vi "复件 SIMCOMCommunicationTool.vi"(6 "Debug":bool=TRUE, 7 "MEID":string, 8 "error in":errorcluster, 9 "DelayTime":u32=100, 10 "通信协议名称":string, 11 "VISA资源名称":refnum<visa-resource-name>="COM26") -> (0 "error out":errorcluster, 1 "CMD":string="发送 重启:AT+CRESET\r反馈:\r\nOK\r\n\r\n", 2 "反馈结果":bool=TRUE, 3 "响应":string="\r\nOK\r\n", 4 "ReturnData":string)   [LabVIEW 2013]
doc: "本范例根据用户指示，对串口执行读写操作。范例运行时可按下“写入”或“读取”按钮，以及修改“读数”。\n\n设置的串口参数必须匹配连接仪器或设备的参数。本范例中，“读数”参数可指定串口读取的字节数。如端口字节超过指定的字节数，超出部分将不会被读取。如端口字节数少于指定的字节数，将返回超时错误。\n\n本范例可扩展流控制选项以包括XON和XOFF，从而允许用户选择控制字符。同时，用户可启用或禁用中止符。部分设备需要通过终止符确定命令字符串的结束位置。部分设备将发送终止符以说明待读取数据的末端。本范例演示了缓冲区中检测到终止符时，结束“读取”操作或添加终止符至“写入”数据末端的方法。"
uses:
  <vilib>/Utility/NIReport.llb/NI_report.lvclass
  C:/Program Files/National Instruments/LabVIEW 2013/examples/Instrument IO/Serial/support/Serial - Settings.ctl
  SourceCode/GlobalValue.vi
  <vilib>/Utility/error.llb/Error Cluster From Error Code.vi
  <vilib>/addons/_office/excel.llb/Excel Get Data ([str]).vi
  <vilib>/Instr/_visa.llb/VISA Configure Serial Port (Instr).vi
  <vilib>/ErrorRing/Error Ring.xnode
  <vilib>/addons/_office/NI_ReportGenerationToolkit.lvlib
  <vilib>/Utility/NIReport.llb/Excel/NI_Excel.lvclass
panel:
  out "Data":string[][](array[string])=[["8986031490021881534", "460036161669975", "2A645416CB435F94", "8006A127", "460036161669975@mycdma.cn", "DB60264368A1D188", "18101891253", "A1000021A59070"], ["8986031490021881535", "460036161669976", "32FA5764D69C76BE", "80FAE4E6", "460036161669976@mycdma.cn", "B3AA1B3D2F0D5593", "18964872399", "A1000021A58D61"], ["", "", "", "", "", "", "", ""], ["", "", "", "", "", "", "", ""], ["", "", "", "", "", "", "", ""], ["", "", "", "", "", "", "", ""], ["", "", "", "", "", "", "", ""], ["", "", "", "", "", "", "", ""], ["", "", "", "", "", "", "", ""], ["", "", "", "", "", "", "", ""], ["", "各位，模块烧号主要是写五码，包括IMSI、AKEY、MEID（ESN）、AN(EVDO USER)、AAA(EVDO PWD)。", "", "", "", "", "", ""], ["", "其中ESN和MEID在模块出厂时已经写入，两者均可通过AT指令读取，但ESN不可更改。", "", "", "", "", "", ""], ["", "经询问及实际测试，上海电信绑定ESN号而广东电信未绑定，意味着上海电信五码烧录到其它模块是不可用的，但广东电信则无此限制。", "", "", "", "", "", ""], ["", "", "", "", "", "", "", ""], ["", "", "", "", "", "", "", ""], ["", "目前已确定跟上海电信合作，后续模块及卡号使用过程中，如遇到模块损坏，则意味着该卡必须销号（除非向电信申请绑定新的ESN），否则烧录到其它模块中是没用的。", "", "", "", "", "", ""]]
  in  "命令列表":u16(ring)=18 items=["查询RTRECF", "设置RTRECF", "查询MEID", "设置MEID", "查询ESN", "设置ESN", "查询AKEY", "设置AKEY", "查询IMSI1", "设置IMSI1", "查询IMSI2", "设置IMSI2", "查询IMSI3", "设置IMSI3", "设置EVDO账号", "设置EVDO密码", "打开音频LOOPBACK", "关闭音频LOOPBACK", "重启"]
  out "ConfigPath":string="D:\\导航\\T-BOX\\新建文件夹\\config\\通信协议.xls"
  out "DataType":string="AT+CRESET"
  out "命令":string="AT+CRESET\r"
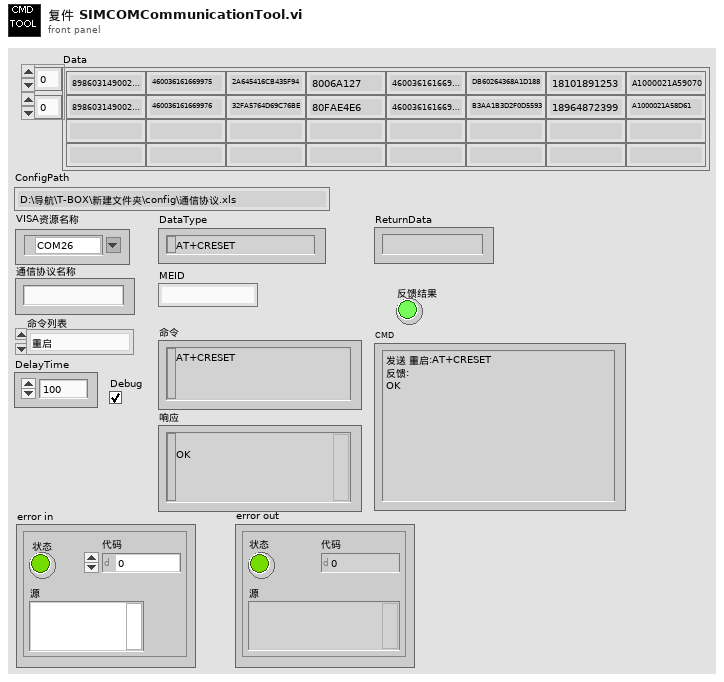
[diagram p1: front panel]
types:
  T1 = enum32{"invalid app kind", "Development System", "Run Time System", "Student Edition", "Embedded LabVIEW", "Evaluation", "Custom"}
  T2 = enum16{"maximized", "minimized", "normal", "no change"}
  T3 = enum16{"Standard Report", "HTML", "Word", "Excel"}
  T4 = typedef "Serial - Settings.ctl" = cluster{"波特率":u32, "数据比特":u16, "奇偶":enum16{"None", "Odd", "Even", "Mark", "Space"}, "停止位":u16, "流控制":u16}
  T5 = cluster{"IMSI":string, "AKEY":string, "ESN":string, "EVDO账号":string, "EVDO密码":string}
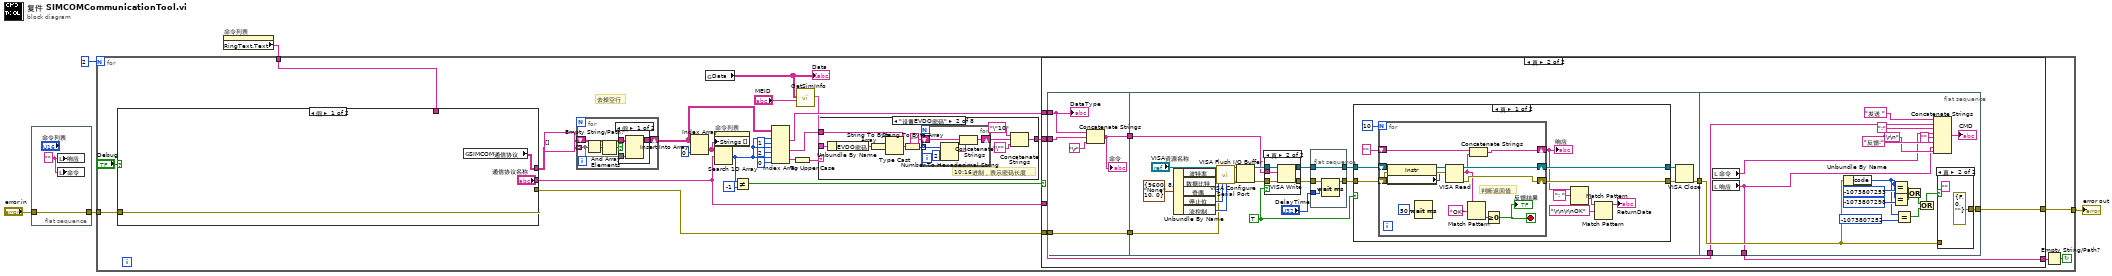
[diagram p0: block diagram]
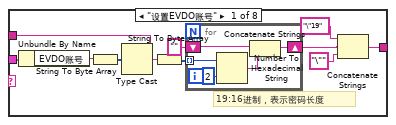
[diagram p3: hidden frame]
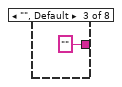
[diagram p4: hidden frame]
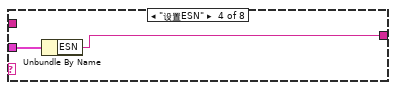
[diagram p5: hidden frame]
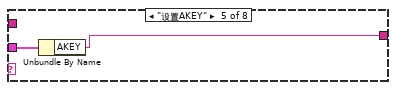
[diagram p6: hidden frame]
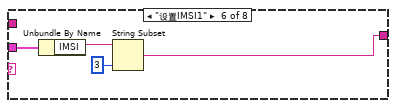
[diagram p7: hidden frame]
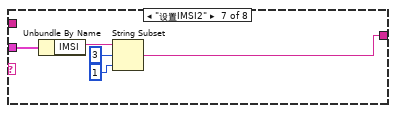
[diagram p8: hidden frame]
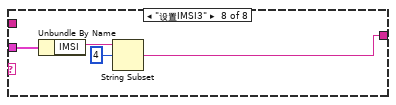
[diagram p9: hidden frame]
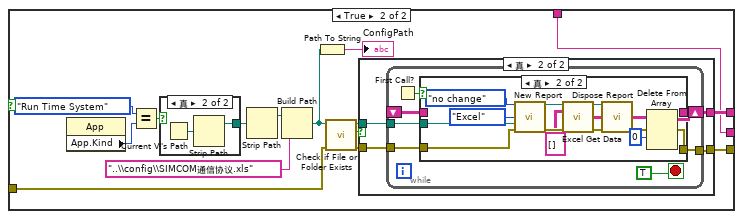
[diagram p10: hidden frame]
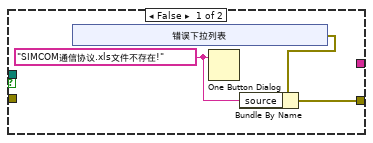
[diagram p11: hidden frame]
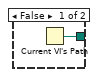
[diagram p13: hidden frame]
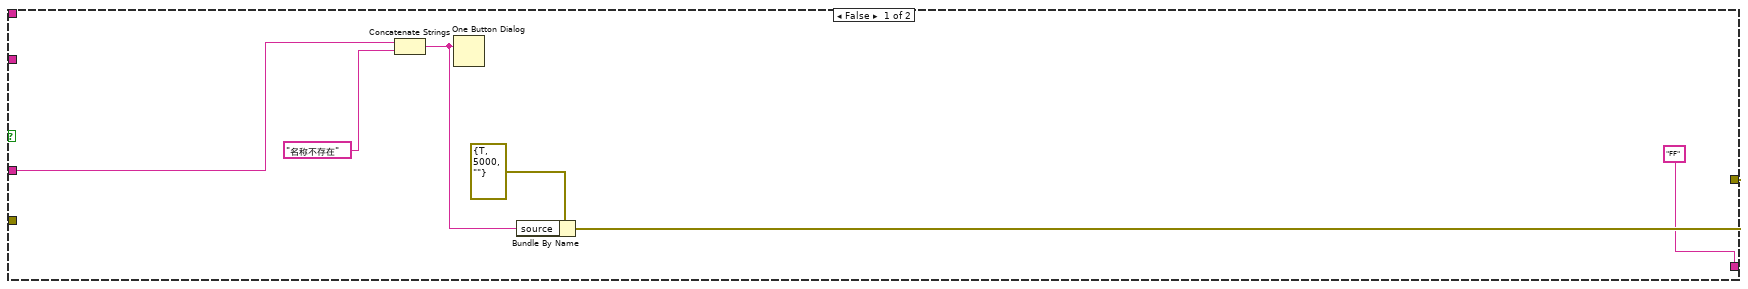
[diagram p14: hidden frame]
diagram:
  n1 = flat-sequence {
    tunnel: "error in" -> [w6]
    tunnel: [w6] -> w2
    frame #0 {
      w7 = "" ("响应")
      n2 = local write "响应"(w7) -> ()
      n3 = local write "命令"(w7) -> ()
    }
  }
  n4 = property on="命令列表" class="Ring (严格)"() -> ("RingText.Text"=w1:string)  [unwired: 2 in, 2 out]
  n5 = for {
    N: 2 -> [_]
    tunnel: w2 -> [w22]
    tunnel: [w34] -> w5
    tunnel: w1 -> [w14]
    stop <- w20 continue-if-true
    # "去掉空行"
    n6 = case shown="假" "Debug" {
      tunnel: [w93 w98] -> w33
      tunnel: w22 -> [w93 w97]
      tunnel: ["通信协议名称" w95] -> w26
      tunnel: [w92 w96] -> w16
      tunnel: w14 -> [_ w95]
      frame False {
        n7 = global read "GlobalValue.vi" "SIMCOM通信协议"() -> (w92:string[][])
      }
      frame True {
        n8 = property class="App"() -> ("App.Kind"=w107:T1)  [unwired: 2 in, 2 out]
        n9 = Equal?(x=T1."Run Time System" ("y"), y=w107) -> (x = y?=w109:bool)
        n10 = case shown="真" w109 {
          tunnel: [w143 w145] -> w108
          frame False {
            n11 = Current VI's Path() -> (path=w143:path)
          }
          frame True {
            n12 = Current VI's Path() -> (path=w144:path)
            n13 = Strip Path(path=w144) -> (stripped path=w145:path)  [unwired: 1 out]
          }
        }
        n14 = Strip Path(path=w108) -> (stripped path=w102:path)  [unwired: 1 out]
        n15 = Build Path(base path=w102, name or relative path="..\\config\\SIMCOM通信协议.xls" ("连接的字符串")) -> (appended path=w104:path)
        n16 = Path To String(path=w104) -> (string=→"ConfigPath":string)
        n17 = call <vilib>:"Check if File or Folder Exists.vi"("error in (no error)"=w97, "path"=w104) -> ("error out"=w99:errorcluster, "file or folder exists?"=w101:bool, "dup path"=w100:path)  [unwired: 7 out]
        n18 = case shown="真" w101 {
          tunnel: w100 -> [_ w120]
          tunnel: w99 -> [_ w119]
          tunnel: [w111 w118] -> w98
          tunnel: [_ w117] -> w96
          frame False {
            w112 = "SIMCOM通信协议.xls文件不存在!" ("消息")
            n19 = xnode "错误下拉列表"() -> ("错误输出"=w110:errorcluster)
            n20 = One Button Dialog(message=w112) -> ()  [unwired: 1 in, 1 out]
            n21 = Bundle By Name(cluster=w110, "source"=w112) -> (w111:errorcluster)
          }
          frame True {
            n22 = while {
              tunnel: w120 -> [w126]
              tunnel: [w125] -> w118
              tunnel: w119 -> [w124]
              shift-right: [w127] -> w117
              shift-left: _ -> [w122]
              stop <- TRUE stop-if-true
              n23 = First Call?() -> (First Call?: T/F=w121:bool)
              n24 = case shown="真" w121 {
                tunnel: [w129 w133] -> w127
                tunnel: w126 -> [_ w132]
                tunnel: [w128 w131] -> w125
                tunnel: w124 -> [w128 w130]
                tunnel: w122 -> [w129 _]
                frame False {
                }
                frame True {
                  n25 = call <vilib>:"New Report.vi"("window state (normal)"=T2."no change", "report type"=T3."Excel", "template (empty)"=w132, "error in (no error)"=w130) -> ("report out"=w138:refnum<class "NI_report.lvclass">, "error out"=w139:errorcluster)  [unwired: 2 in, 8 out]
                  n26 = call-poly <vilib>:"Excel Get Data.vi"("report in"=w138, "data type"=string[][] [], "error in (no error)"=w139) -> ("report out"=w135:refnum<class "NI_report.lvclass">, "data"=w140:string[][], "error out"=w134:errorcluster)  [unwired: 10 in]
                  n27 = call-dynamic "Dispose Report.vi"("report in"=w135, "error in (no error)"=w134) -> ("error out"=w131:errorcluster)  [unwired: 3 in, 10 out]
                  n28 = Delete From Array(array=w140, index (row)=0 ("索引 (行)")) -> (array with subset deleted=w133:string[][])  [unwired: 2 in, 1 out]
                }
              }
            }
          }
        }
      }
    }
    n29 = for {
      tunnel: w16 -> [w35] mode=indexing
      shift-right: [w38] -> w15
      shift-left: string[][] [] -> [w39]
      n30 = Empty String/Path?(string/path=w35) -> (empty?=w37:bool[])
      n31 = And Array Elements(Boolean array=w37) -> (logical AND=w36:bool)
      n32 = case shown="假" w36 {
        tunnel: w39 -> [w42 w43]
        tunnel: [w41 w43] -> w38
        tunnel: w35 -> [w40 _]
        frame False {
          n33 = Insert Into Array(array=w42, new element=w40) -> (w41:string[][])  [unwired: 2 in]
        }
        frame True {
        }
      }
    }
    n34 = Index Array(array=w15, index (col)=0 ("禁用的索引 (列)")) -> (element=w24:string[])  [unwired: 1 in]
    n35 = global read "GlobalValue.vi" "Data"() -> (w9:string[][])
    "Data" <- w9
    n36 = property on="命令列表" class="Ring (严格)"("Strings []"=w24) -> ()  [unwired: 2 in, 2 out]
    n37 = Search 1D Array(1D array=w24, element=w26) -> (index of element=w19:i32)  [unwired: 1 in]
    n38 = Not Equal?(x=w19, y=-1) -> (x != y?=w28:bool)
    n39 = Index Array(array=w15, index (row) #1=w19, index (col) #1=1 ("索引 (列)"), index (row) #2=w19, index (col) #2=2 ("索引 (列)"), index (row) #3=w19, index (col) #3=0 ("索引 (列)")) -> (element #1=w12:string, element #2=w8:string, element #3=w13:string)
    n40 = To Upper Case(1:w13) -> (0:w18:string)
    n41 = call "GetSimInfo.vi"("MEID"="MEID", "Data"=w9) -> ("SIMInfo"=w10:T5)  [unwired: 9 in]
    n42 = case shown="\"设置EVDO密码\"" w18 {
      tunnel: [w47 w62 "" w75 w77 w79 w84 w89] -> w27
      tunnel: w10 -> [w46 w60 _ w76 w78 w82 w87 w91]
      tunnel: w8 -> [w44 w59 _ _ _ _ _ _]
      frame "设置EVDO账号" {
        # "19:16进制，表示密码长度"
        n43 = Unbundle By Name(w46) -> ("EVDO账号"=w45:string)
        n44 = String To Byte Array(string=w45) -> (unsigned byte array=w53:u8[])
        n45 = Type Cast(x=w53) -> ()  [unwired: 1 in, 1 out]
        n46 = String To Byte Array(string=w44) -> (unsigned byte array=w52:u8[])
        n47 = for {
          tunnel: w52 -> [w58] mode=indexing
          shift-right: [w56] -> w48
          shift-left: "" -> [w55]
          n48 = Number To Hexadecimal String(1:i16 2 ("宽度(-)"), 2:w58) -> (0:w57:string)
          n49 = Concatenate Strings(w55, w57) -> (w56:string)
        }
        n50 = Concatenate Strings("\"19" ("字符串"), w48, "\"" ("字符串")) -> (w47:string)
      }
      frame "设置EVDO密码" {
        # "10:16进制，表示密码长度"
        n51 = Unbundle By Name(w60) -> ("EVDO密码"=w61:string)
        n52 = String To Byte Array(string=w61) -> (unsigned byte array=w68:u8[])
        n53 = Type Cast(x=w68) -> ()  [unwired: 1 in, 1 out]
        n54 = String To Byte Array(string=w59) -> (unsigned byte array=w67:u8[])
        n55 = for {
          tunnel: w67 -> [w73] mode=indexing
          shift-right: [w71] -> w65
          shift-left: "" -> [w70]
          n56 = Number To Hexadecimal String(1:i16 2 ("宽度(-)"), 2:w73) -> (0:w72:string)
          n57 = Concatenate Strings(w70, w72) -> (w71:string)
        }
        n58 = Concatenate Strings("\"10" ("字符串"), w65, "\"" ("字符串")) -> (w62:string)
      }
      frame "", Default {
      }
      frame "设置ESN" {
        n59 = Unbundle By Name(w76) -> ("ESN"=w75:string)
      }
      frame "设置AKEY" {
        n60 = Unbundle By Name(w78) -> ("AKEY"=w77:string)
      }
      frame "设置IMSI1" {
        n61 = Unbundle By Name(w82) -> ("IMSI"=w81:string)
        n62 = String Subset(string=w81, length (rest)=3 ("长度（剩余）")) -> (substring=w79:string)  [unwired: 1 in]
      }
      frame "设置IMSI2" {
        n63 = Unbundle By Name(w87) -> ("IMSI"=w86:string)
        n64 = String Subset(string=w86, offset (0)=3 ("偏移量(0)"), length (rest)=1 ("长度（剩余）")) -> (substring=w84:string)
      }
      frame "设置IMSI3" {
        n65 = Unbundle By Name(w91) -> ("IMSI"=w90:string)
        n66 = String Subset(string=w90, offset (0)=4 ("偏移量(0)")) -> (substring=w89:string)  [unwired: 1 in]
      }
    }
    n67 = case shown="真" w28 {
      tunnel: w26 -> [w151 w152]
      tunnel: w12 -> [_ w160]
      tunnel: w27 -> [_ w159]
      tunnel: w33 -> [_ w158]
      tunnel: [w147 w156] -> w34
      tunnel: ["FF" ("响应") w154] -> w21
      frame False {
        n68 = Concatenate Strings(w151, "名称不存在" ("消息")) -> (w148:string)
        n69 = One Button Dialog(message=w148) -> ()  [unwired: 1 in, 1 out]
        n70 = Bundle By Name(cluster=errorcluster {"status"=TRUE, "code"=5000, "source"=""} ("error in 1 (no error)"), "source"=w148) -> (w147:errorcluster)
      }
      frame True {
        n71 = flat-sequence {
          tunnel: w160 -> [w164]
          tunnel: w159 -> [w163]
          tunnel: w158 -> [w165]
          tunnel: [w165] -> w157
          tunnel: [w162] -> w153
          tunnel: w157 -> [w174]
          tunnel: [w173] -> w155
          tunnel: w153 -> [w167]
          tunnel: [w238] -> w156
          tunnel: w155 -> [w237]
          tunnel: w152 -> [w234]
          tunnel: [w226] -> w154
          frame #0 {
            n72 = Concatenate Strings(w164, w163, "\r") -> (w162:string)
            "命令" <- w162
            "DataType" <- w164
          }
          frame #1 {
            w166 = TRUE
            n73 = Unbundle By Name(T4 {"波特率"=9600, "数据比特"=8, "奇偶"=enum."None", "停止位"=10, "流控制"=0} ("串口设置")) -> ("波特率"=w183:u32, "数据比特"=w184:u16, "奇偶"=w185:enum16{"None", "Odd", "Even", "Mark", "Space"}, "停止位"=w186:u16, "流控制"=w179:u16)
            n74 = call-poly "VISA Configure Serial Port"("VISA resource name"="VISA资源名称", "baud rate (9600)"=w183, "data bits (8)"=w184, "parity (0:none)"=w185, "error in (no error)"=w174, "stop bits (10: 1 bit)"=w186, "flow control (0:none)"=w179) -> ("VISA resource name out"=w171:refnum<visa-resource-name>, "error out"=w172:errorcluster)  [unwired: 3 in, 4 out]
            n75 = VISA Flush I/O Buffer(VISA resource name=w171, error in (no error)=w172) -> (VISA resource name out=w170:refnum<visa-resource-name>, error out=w168:errorcluster)  [unwired: 1 in]
            n76 = case shown="真" w166 {
              tunnel: w170 -> [w192 w197]
              tunnel: [w192 w196] -> w178
              tunnel: [w191 w195] -> w177
              tunnel: w168 -> [w191 w194]
              tunnel: w167 -> [_ w193]
              frame False {
              }
              frame True {
                n77 = VISA Write(VISA resource name=w197, write buffer=w193, error in (no error)=w194) -> (VISA resource name out=w196:refnum<visa-resource-name>, error out=w195:errorcluster)  [unwired: 1 out]
              }
            }
            n78 = flat-sequence {
              tunnel: w177 -> [w190]
              tunnel: [w190] -> w175
              tunnel: w178 -> [w189]
              tunnel: [w189] -> w176
              tunnel: "DelayTime" -> [w188]
              frame #0 {
                n79 = Wait (ms)(milliseconds to wait=w188) -> ()  [unwired: 1 out]
              }
            }
            n80 = case shown="真" w166 {
              tunnel: [w207 w224] -> w180
              tunnel: w176 -> [w206 w224]
              tunnel: [w208 w223] -> w181
              tunnel: w175 -> [w205 w223]
              frame True {
                n81 = for {
                  N: 10 -> [_]
                  shift-right: [w222] -> w208
                  shift-left: w205 -> [w216]
                  shift-right: [w214] -> w199
                  shift-left: "" ("read buffer") -> [w215]
                  shift-right: [w221] -> w207
                  shift-left: w206 -> [w217]
                  stop <- w209 stop-if-true
                  # "判断返回值"
                  n82 = property class="Instr"(reference=w217, error in=w216) -> (reference out=w220:refnum<visa-resource-name>, error out=w219:errorcluster, "Serial Settings:Number of Bytes at Serial Port"=w218:u32)
                  n83 = Wait (ms)(milliseconds to wait=u32 50 ("等待时间（毫秒）")) -> ()  [unwired: 1 out]
                  n84 = VISA Read(VISA resource name=w220, byte count=w218, error in (no error)=w219) -> (VISA resource name out=w221:refnum<visa-resource-name>, read buffer=w212:string, error out=w222:errorcluster)  [unwired: 1 out]
                  n85 = Match Pattern(string=w212, regular expression="OK" ("正则表达式")) -> (offset past match=w213:i32)  [unwired: 1 in, 3 out]
                  n86 = Concatenate Strings(w215, w212) -> (w214:string)
                  n87 = Greater Or Equal To 0?(x=w213) -> (x >= 0?=w209:bool)
                  "反馈结果" <- w209
                }
                "响应" <- w199
                n88 = Match Pattern(string=w199, regular expression=": " ("正则表达式")) -> (after substring=w200:string)  [unwired: 1 in, 3 out]
                n89 = Match Pattern(string=w200, regular expression="\r\n\r\nOK" ("正则表达式")) -> (before substring=→"ReturnData":string)  [unwired: 1 in, 3 out]
              }
              frame False {
              }
            }
            n90 = VISA Close(VISA resource name=w180, error in (no error)=w181) -> (error out=w173:errorcluster)
          }
          frame #2 {
            n91 = local read "命令"() -> (w227:string)
            n92 = local read "响应"() -> (w226:string)
            n93 = Unbundle By Name(w237) -> ("code"=w233:i32)
            n94 = Equal?(x=w233, y=-1073807253) -> (x = y?=w235:bool)
            n95 = Equal?(x=w233, y=-1073807298) -> (x = y?=w231:bool)
            n96 = Equal?(x=w233, y=-1073807252) -> (x = y?=w228:bool)
            n97 = Or(x=w235, y=w231) -> (x .or. y?=w229:bool)
            n98 = Or(x=w229, y=w228) -> (x .or. y?=w230:bool)
            n99 = Concatenate Strings("发送 " ("字符串"), w234, ":" ("字符串"), w227, "" ("字符串"), "反馈:" ("字符串"), w226, "\r\n") -> (→"CMD":string)
            n100 = case shown="真" w230 {
              tunnel: [w245 errorcluster {"status"=FALSE, "code"=0, "source"=""} ("t")] -> w238
              tunnel: w237 -> [w245 _]
              frame False {
              }
              frame True {
                (unwired) ""
              }
            }
          }
        }
      }
    }
    n101 = Empty String/Path?(string/path=w21) -> (empty?=w20:bool)
  }
  "error out" <- w5
